vi "TEST - Index Array Elements.vi"(8 "error in (no error)":errorcluster) -> (0 "error out":errorcluster, 2 "Pass?":bool)   [LabVIEW 2020]
doc: "This VI template can be used for the functional testing of VIs; this implementation includes handling for the testing of polymorphic VIs, and the polymorphic elements should be removed if not needed.\n\nCoded by Douglas A. Femec, January 24, 2006.\n\nCopyright (c) 2005-2006 MKS Instruments, Inc.\nAll rights reserved."
uses:
  TEST - Index Array Elements - Inputs.ctl
  Polymorphizer+ Data Type.ctl
  TEST - Index Array Elements - Outputs.ctl
  source/library/Index Array Elements/Index 1D Array Elements (EXT).vi
  source/library/Index Array Elements/Index 1D Array Elements (I64).vi
  source/library/Index Array Elements/Index 1D Array Elements (U64).vi
  source/library/Index Array Elements/Index 1D Array Elements (LVObject).vi
  source/library/Index Array Elements/Index 1D Array Elements (DBL).vi
  source/library/Index Array Elements/Index 1D Array Elements (SGL).vi
  source/library/Index Array Elements/Index 1D Array Elements (I32).vi
  source/library/Index Array Elements/Index 1D Array Elements (I16).vi
  source/library/Index Array Elements/Index 1D Array Elements (I8).vi
  source/library/Index Array Elements/Index 1D Array Elements (U32).vi
  source/library/Index Array Elements/Index 1D Array Elements (U16).vi
  source/library/Index Array Elements/Index 1D Array Elements (U8).vi
  source/library/Index Array Elements/Index 1D Array Elements (CXT).vi
  source/library/Index Array Elements/Index 1D Array Elements (CDB).vi
  source/library/Index Array Elements/Index 1D Array Elements (CSG).vi
  source/library/Index Array Elements/Index 1D Array Elements (Boolean).vi
  source/library/Index Array Elements/Index 1D Array Elements (String).vi
  source/library/Index Array Elements/Index 1D Array Elements (Path).vi
  source/library/Index Array Elements/Index 1D Array Elements (Variant).vi
  source/library/openg_array.lvlib
  TestClass/TestClass.lvclass
panel:
  out "Generated Outputs":T1[][](array[typedef])=[[{"Description"="Expect empty array", "Elements"=[]}, {"Description"="Expect empty array", "Elements"=[]}, {"Description"="Expect empty array", "Elements"=[]}, {"Description"="Expect empty array", "Elements"=[]}, {"Description"="Expect empty array", "Elements"=[]}, {"Description"="Expect empty array", "Elements"=[]}, {"Description"="Expect empty array", "Elements"=[]}, {"Description"="Expect empty array", "Elements"=[]}, {"Description"="Expect empty array", "Elements"=[]}, {"Description"="Expect empty array", "Elements"=[]}, {"Description"="Expect empty array", "Elements"=[]}, {"Description"="Expect empty array", "Elements"=[]}, {"Description"="Expect empty array", "Elements"=[]}, {"Description"="Expect empty array", "Elements"=[]}, {"Description"="Expect empty array", "Elements"=[]}, {"Description"="Expect empty array", "Elements"=[]}], [{"Description"="Expect no elements filtered", "Elements"=[]}, {"Description"="Expect no elements filtered", "Elements"=[]}, {"Description"="Expect no elements filtered", "Elements"=[]}, {"Description"="Expect no elements filtered", "Elements"=[]}, {"Description"="Expect no elements filtered", "Elements"=[]}, {"Description"="Expect no elements filtered", "Elements"=[]}, {"Description"="Expect no elements filtered", "Elements"=[]}, {"Description"="Expect no elements filtered", "Elements"=[]}, {"Description"="Expect no elements filtered", "Elements"=[]}, {"Description"="Expect no elements filtered", "Elements"=[]}, {"Description"="Expect no elements filtered", "Elements"=[]}, {"Description"="Expect no elements filtered", "Elements"=[]}, {"Description"="Expect no elements filtered", "Elements"=[]}, {"Description"="Expect no elements filtered", "Elements"=[]}, {"Description"="Expect no elements filtered", "Elements"=[]}, {"Description"="Expect no elements filtered", "Elements"=[]}], [{"Description"="Expect some elements", "Elements"=[1.0, 5.0]}, {"Description"="Expect some elements", "Elements"=[1.0, 5.0]}, {"Description"="Expect some elements", "Elements"=[1.0, 5.0]}, {"Description"="Expect some elements", "Elements"=[1.0, 5.0]}, {"Description"="Expect some elements", "Elements"=[1.0, 5.0]}, {"Description"="Expect some elements", "Elements"=[1.0, 5.0]}, {"Description"="Expect some elements", "Elements"=[1.0, 5.0]}, {"Description"="Expect some elements", "Elements"=[1.0, 5.0]}, {"Description"="Expect some elements", "Elements"=[1.0, 5.0]}, {"Description"="Expect some elements", "Elements"=[1.0, 5.0]}, {"Description"="Expect some elements", "Elements"=[1.0, 5.0]}, {"Description"="Expect some elements", "Elements"=[1.0, 5.0]}, {"Description"="Expect some elements", "Elements"=[1.0, 5.0]}, {"Description"="Expect some elements", "Elements"=[1.0, 5.0]}, {"Description"="Expect some elements", "Elements"=[1.0, 5.0]}, {"Description"="", "Elements"=[]}], [{"Description"="Expect all elements filtered", "Elements"=[0.0, 1.0]}, {"Description"="Expect all elements filtered", "Elements"=[0.0, 1.0]}, {"Description"="Expect all elements filtered", "Elements"=[0.0, 1.0]}, {"Description"="Expect all elements filtered", "Elements"=[0.0, 1.0]}, {"Description"="Expect all elements filtered", "Elements"=[0.0, 1.0]}, {"Description"="Expect all elements filtered", "Elements"=[0.0, 1.0]}, {"Description"="Expect all elements filtered", "Elements"=[0.0, 1.0]}, {"Description"="Expect all elements filtered", "Elements"=[0.0, 1.0]}, {"Description"="Expect all elements filtered", "Elements"=[0.0, 1.0]}, {"Description"="Expect all elements filtered", "Elements"=[0.0, 1.0]}, {"Description"="Expect all elements filtered", "Elements"=[0.0, 1.0]}, {"Description"="Expect all elements filtered", "Elements"=[0.0, 1.0]}, {"Description"="Expect all elements filtered", "Elements"=[0.0, 1.0]}, {"Description"="Expect all elements filtered", "Elements"=[0.0, 1.0]}, {"Description"="Expect all elements filtered", "Elements"=[0.0, 1.0]}, {"Description"="Expect all elements filtered", "Elements"=[0.0, 1.0]}]] {"Elements" format="%.2f"}
  in  "Expected Outputs":T1[](array[typedef])=[{"Description"="Expect empty array", "Elements"=[]}, {"Description"="Expect no elements filtered", "Elements"=[]}, {"Description"="Expect some elements", "Elements"=[1.0, 5.0]}, {"Description"="Reverse Elements", "Elements"=[0.0, 2.0, 4.0, 6.0]}] {"Elements" format="%.2f"}
  in  "Inputs":T2[](array[typedef])=[{"Description"="Empty arrays", "Data Types to Test"=[enum."EXT", enum."DBL", enum."SGL", enum."I32", enum."I16", enum."I8", enum."U32", enum."U16", enum."U8", enum."CXT", enum."CDB", enum."CSG", enum."Boolean", enum."String", enum."Path", enum."Variant", enum."I64", enum."U64", enum."LabVIEW Object"], "Array"=[], "Indices"=[]}, {"Description"="No element to filter", "Data Types to Test"=[enum."EXT", enum."DBL", enum."SGL", enum."I32", enum."I16", enum."I8", enum."U32", enum."U16", enum."U8", enum."CXT", enum."CDB", enum."CSG", enum."Boolean", enum."String", enum."Path", enum."Variant", enum."I64", enum."U64", enum."LabVIEW Object"], "Array"=[0.0, 0.0, 0.0, 0.0], "Indices"=[]}, {"Description"="Get some elements", "Data Types to Test"=[enum."EXT", enum."DBL", enum."SGL", enum."I32", enum."I16", enum."I8", enum."U32", enum."U16", enum."U8", enum."CXT", enum."CDB", enum."CSG", enum."String", enum."Path", enum."Variant", enum."I64", enum."U64", enum."LabVIEW Object"], "Array"=[1.0, 3.0, 5.0, 7.0], "Indices"=[0, 2]}, {"Description"="Reverse Elements", "Data Types to Test"=[enum."EXT", enum."DBL", enum."SGL", enum."I32", enum."I16", enum."I8", enum."U32", enum."U16", enum."U8", enum."CXT", enum."CDB", enum."CSG", enum."String", enum."Path", enum."Variant", enum."I64", enum."U64", enum."LabVIEW Object"], "Array"=[6.0, 4.0, 2.0, 0.0], "Indices"=[3, 2, 1, 0]}] {"Array" format="%.2f"}
  # "Copyright (c) 2005-2006 MKS Instruments, Inc.\nAll rights reserved."
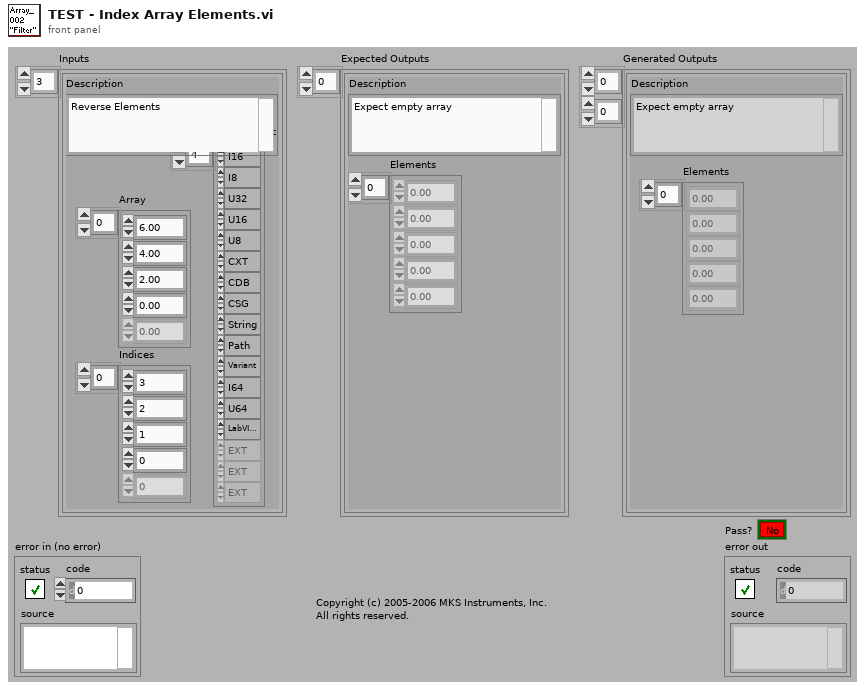
[diagram p1: front panel]
types:
  T1 = typedef "TEST - Index Array Elements - Outputs.ctl" = cluster{"Description":string, "Elements":sgl[]}
  T2 = typedef "TEST - Index Array Elements - Inputs.ctl" = cluster{"Description":string, "Data Types to Test":T3[], "Array":sgl[], "Indices":i32[]}
  T3 = typedef "Polymorphizer+ Data Type.ctl" = enum16{"EXT", "DBL", "SGL", "I32", "I16", "I8", "U32", "U16", "U8", "CXT", "CDB", "CSG", "Boolean", "String", "Path", "Variant", "CTL-REF", "GEN-REF", "GObj-REF", "VI-REF", "ENUM", "ERR", "FILE-REF", "MENU-REF", "MENU-RING", "PICT-RING", "TXT&PICT-RING", "TXT-RING", "I64", "U64", "LabVIEW Object"}
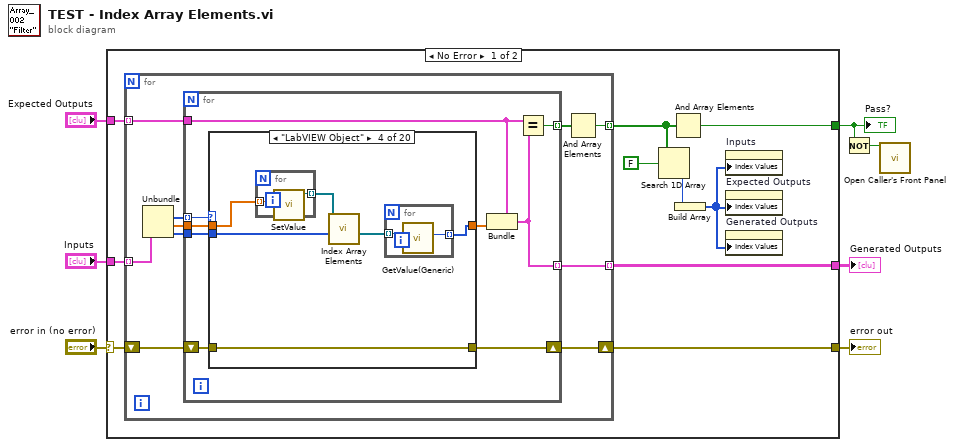
[diagram p0: block diagram]
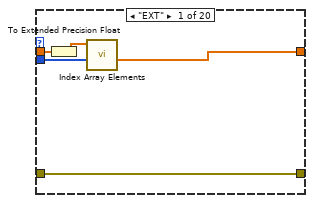
[diagram p2: hidden frame]
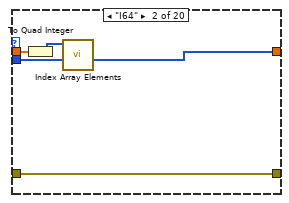
[diagram p3: hidden frame]
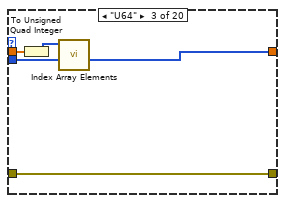
[diagram p4: hidden frame]
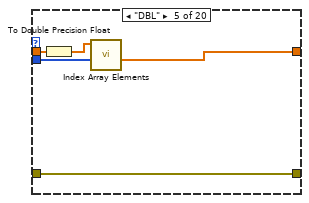
[diagram p5: hidden frame]
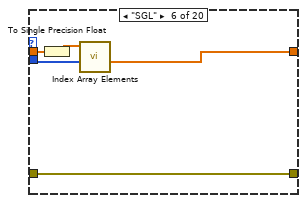
[diagram p6: hidden frame]
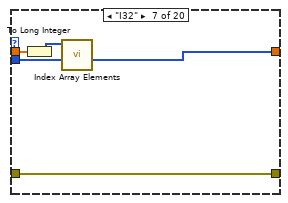
[diagram p7: hidden frame]
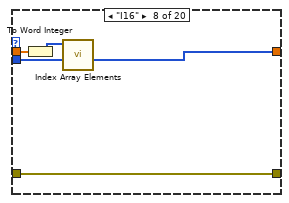
[diagram p8: hidden frame]
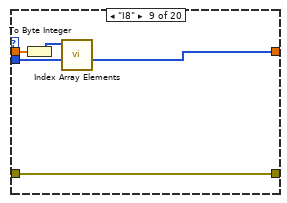
[diagram p9: hidden frame]
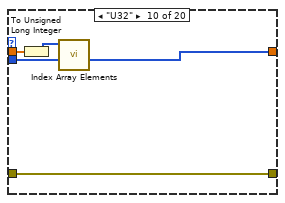
[diagram p10: hidden frame]
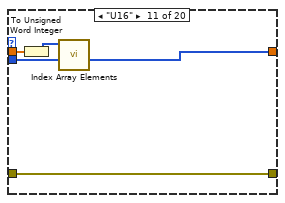
[diagram p11: hidden frame]
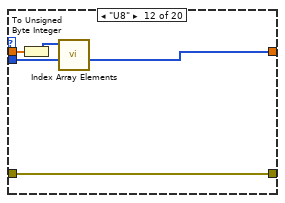
[diagram p12: hidden frame]
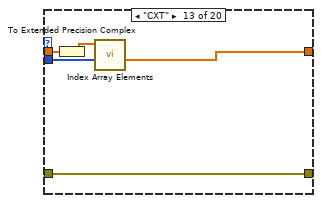
[diagram p13: hidden frame]
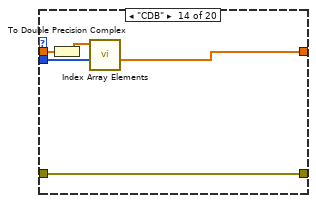
[diagram p14: hidden frame]
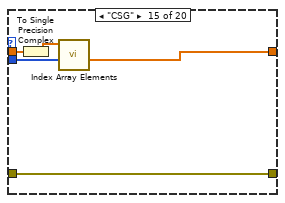
[diagram p15: hidden frame]
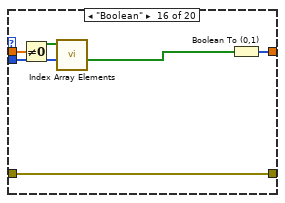
[diagram p16: hidden frame]
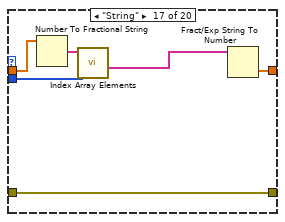
[diagram p17: hidden frame]
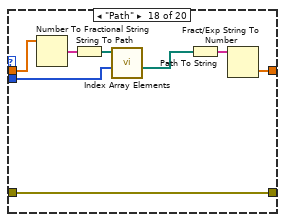
[diagram p18: hidden frame]
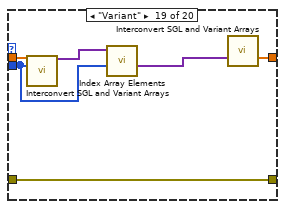
[diagram p19: hidden frame]
diagram:
  n1 = case shown="No Error" "error in (no error)" {
    selector: "error in (no error)" -> [w16 w145]
    tunnel: [w17 w145] -> w6
    tunnel: "Expected Outputs" -> [w14 _]
    tunnel: "Inputs" -> [w15 _]
    tunnel: [w13 _] -> w3
    tunnel: [w12 _] -> w2
    frame No Error {
      n2 = for {
        shift-right: [w22] -> w17
        shift-left: w16 -> [w23]
        tunnel: w15 -> [w24] mode=indexing
        tunnel: w14 -> [w27] mode=indexing
        tunnel: [w26] -> w13 mode=indexing
        tunnel: [w21] -> w11 mode=indexing
        n3 = Unbundle(w24) -> ("Data Types to Test"=w20:T3[], "Array"=w18:sgl[], "Indices"=w19:i32[])  [unwired: 1 out]
        n4 = for {
          tunnel: w27 -> [w36]
          tunnel: [w34] -> w26 mode=indexing
          tunnel: [w35] -> w25 mode=indexing
          shift-right: [w29] -> w22
          shift-left: w23 -> [w30]
          tunnel: w20 -> [w31] mode=indexing
          tunnel: w18 -> [w33]
          tunnel: w19 -> [w32]
          n5 = case shown="\"LabVIEW Object\"" w31 {
            tunnel: w33 -> [w41 w46 w51 w55 w66 w71 w76 w81 w86 w91 w96 w101 w106 w111 w116 w122 w128 w135 w141 w143]
            tunnel: [w39 w44 w49 w52 w64 w69 w74 w79 w84 w89 w94 w99 w104 w109 w114 w121 w127 w134 w139 w143] -> w28
            tunnel: w32 -> [w37 w42 w47 w56 w63 w67 w73 w78 w83 w88 w93 w98 w103 w108 w113 w117 w124 w130 w138 _]
            tunnel: w30 -> [w40 w45 w50 w57 w65 w70 w75 w80 w85 w90 w95 w100 w105 w110 w115 w120 w126 w132 w142 w144]
            tunnel: [w40 w45 w50 w57 w65 w70 w75 w80 w85 w90 w95 w100 w105 w110 w115 w120 w126 w132 w142 w144] -> w29
            frame "EXT" {
              n6 = To Extended Precision Float(1:w41) -> (0:w38:ext[])
              n7 = call-poly "Index Array Elements.vi"("indices"=w37, "array"=w38) -> ("elements"=w39:ext[])  [unwired: 9 in]
            }
            frame "I64" {
              n8 = To Quad Integer(1:w46) -> (0:w43:i64[])
              n9 = call-poly "Index Array Elements.vi"("indices"=w42, "array"=w43) -> ("elements"=w44:i64[])  [unwired: 9 in]
            }
            frame "U64" {
              n10 = To Unsigned Quad Integer(1:w51) -> (0:w48:u64[])
              n11 = call-poly "Index Array Elements.vi"("indices"=w47, "array"=w48) -> ("elements"=w49:u64[])  [unwired: 9 in]
            }
            frame "LabVIEW Object" {
              n12 = for {
                tunnel: w55 -> [w61] mode=indexing
                tunnel: [w60] -> w54 mode=indexing
                n13 = call "SetValue.vi"("Value"=w61) -> ("TestClass out"=w60:refnum<class "TestClass.lvclass">)  [unwired: 9 in, 1 out]
              }
              n14 = call-poly "Index Array Elements.vi"("indices"=w56, "array"=w54) -> ("elements"=w53:refnum<class>[])  [unwired: 9 in]
              n15 = for {
                tunnel: w53 -> [w59] mode=indexing
                tunnel: [w58] -> w52 mode=indexing
                n16 = call "GetValue(Generic).vi"("TestClass in"=w59) -> ("Value"=w58:i32)  [unwired: 8 in, 2 out]
              }
            }
            frame "DBL" {
              n17 = To Double Precision Float(number=w66) -> (double precision float=w62:dbl[])
              n18 = call-poly "Index Array Elements.vi"("indices"=w63, "array"=w62) -> ("elements"=w64:dbl[])  [unwired: 9 in]
            }
            frame "SGL" {
              n19 = To Single Precision Float(number=w71) -> (single precision float=w68:sgl[])
              n20 = call-poly "Index Array Elements.vi"("indices"=w67, "array"=w68) -> ("elements"=w69:sgl[])  [unwired: 9 in]
            }
            frame "I32" {
              n21 = To Long Integer(number=w76) -> (32bit integer=w72:i32[])
              n22 = call-poly "Index Array Elements.vi"("indices"=w73, "array"=w72) -> ("elements"=w74:i32[])  [unwired: 9 in]
            }
            frame "I16" {
              n23 = To Word Integer(number=w81) -> (16bit integer=w77:i16[])
              n24 = call-poly "Index Array Elements.vi"("indices"=w78, "array"=w77) -> ("elements"=w79:i16[])  [unwired: 9 in]
            }
            frame "I8" {
              n25 = To Byte Integer(number=w86) -> (8bit integer=w82:i8[])
              n26 = call-poly "Index Array Elements.vi"("indices"=w83, "array"=w82) -> ("elements"=w84:i8[])  [unwired: 9 in]
            }
            frame "U32" {
              n27 = To Unsigned Long Integer(number=w91) -> (unsigned 32bit integer=w87:u32[])
              n28 = call-poly "Index Array Elements.vi"("indices"=w88, "array"=w87) -> ("elements"=w89:u32[])  [unwired: 9 in]
            }
            frame "U16" {
              n29 = To Unsigned Word Integer(number=w96) -> (unsigned 16bit integer=w92:u16[])
              n30 = call-poly "Index Array Elements.vi"("indices"=w93, "array"=w92) -> ("elements"=w94:u16[])  [unwired: 9 in]
            }
            frame "U8" {
              n31 = To Unsigned Byte Integer(number=w101) -> (unsigned 8bit integer=w97:u8[])
              n32 = call-poly "Index Array Elements.vi"("indices"=w98, "array"=w97) -> ("elements"=w99:u8[])  [unwired: 9 in]
            }
            frame "CXT" {
              n33 = To Extended Precision Complex(1:w106) -> (0:w102:cxt[])
              n34 = call-poly "Index Array Elements.vi"("indices"=w103, "array"=w102) -> ("elements"=w104:cxt[])  [unwired: 9 in]
            }
            frame "CDB" {
              n35 = To Double Precision Complex(1:w111) -> (0:w107:cdb[])
              n36 = call-poly "Index Array Elements.vi"("indices"=w108, "array"=w107) -> ("elements"=w109:cdb[])  [unwired: 9 in]
            }
            frame "CSG" {
              n37 = To Single Precision Complex(1:w116) -> (0:w112:csg[])
              n38 = call-poly "Index Array Elements.vi"("indices"=w113, "array"=w112) -> ("elements"=w114:csg[])  [unwired: 9 in]
            }
            frame "Boolean" {
              n39 = Not Equal To 0?(x=w122) -> (x != 0?=w118:bool[])
              n40 = call-poly "Index Array Elements.vi"("indices"=w117, "array"=w118) -> ("elements"=w119:bool[])  [unwired: 9 in]
              n41 = Boolean To (0,1)(Boolean=w119) -> (0, 1=w121:i16[])
            }
            frame "String" {
              n42 = Number To Fractional String(number=w128) -> (F-format string=w123:string[])  [unwired: 3 in]
              n43 = call-poly "Index Array Elements.vi"("indices"=w124, "array"=w123) -> ("elements"=w125:string[])  [unwired: 9 in]
              n44 = Fract/Exp String To Number(string=w125) -> (number=w127:dbl[])  [unwired: 3 in, 1 out]
            }
            frame "Path" {
              n45 = Number To Fractional String(number=w135) -> (F-format string=w136:string[])  [unwired: 3 in]
              n46 = String To Path(string=w136) -> (path=w129:path[])
              n47 = call-poly "Index Array Elements.vi"("indices"=w130, "array"=w129) -> ("elements"=w131:path[])  [unwired: 9 in]
              n48 = Path To String(path=w131) -> (string=w133:string[])
              n49 = Fract/Exp String To Number(string=w133) -> (number=w134:dbl[])  [unwired: 3 in, 1 out]
            }
            frame "Variant" {
              n50 = call "Interconvert SGL and Variant Arrays.vi"("SGL 1D Array In"=w141, "SGL 1D Array 2 In"=w138) -> ("Variant 1D Array Out"=w137:variant[])  [unwired: 9 in, 4 out]
              n51 = call-poly "Index Array Elements.vi"("indices"=w138, "array"=w137) -> ("elements"=w140:variant[])  [unwired: 9 in]
              n52 = call "Interconvert SGL and Variant Arrays.vi"("Variant 1D Array In"=w140) -> ("SGL 1D Array Out"=w139:sgl[])  [unwired: 10 in, 4 out]
            }
            frame Default {
            }
          }
          n53 = Bundle(cluster=w36, "Elements"=w28) -> (w34:T1)  [unwired: 1 in]
          n54 = Equal?(x=w36, y=w34) -> (x = y?=w35:bool)
        }
        n55 = And Array Elements(Boolean array=w25) -> (logical AND=w21:bool)
      }
      n56 = Search 1D Array(1D array=w11, element=FALSE) -> (index of element=w9:i32)  [unwired: 1 in]
      n57 = And Array Elements(Boolean array=w11) -> (logical AND=w12:bool)
      n58 = Build Array(w9) -> (w8:i32[])
      n59 = property on="Inputs" class="Arr (strict)"("Index Values"=w8) -> ()  [unwired: 2 in, 2 out]
      n60 = property on="Expected Outputs" class="Arr (strict)"("Index Values"=w8) -> ()  [unwired: 2 in, 2 out]
      n61 = property on="Generated Outputs" class="Arr (strict)"("Index Values"=w8) -> ()  [unwired: 2 in, 2 out]
    }
    frame Error {
    }
  }
  "error out" <- w6
  "Pass?" <- w2
  "Generated Outputs" <- w3
  n62 = Not(x=w2) -> (.not. x?=w1:bool)
  n63 = call "Open Caller's Front Panel.vi"("Open?"=w1) -> ()  [unwired: 14 in, 1 out]
